vi "TestKeithley.vi"() -> ()   [LabVIEW 2017]
uses:
  <instrlib>/Keithley 24XX/Public/Data/Read (Measurements).vi
  <instrlib>/Keithley 24XX/Keithley 24XX.lvlib
panel:
  out "Waveform Chart 2":sgl[](graph)
  in  "stop":bool
  out "Current Measurements":sgl[](array[numeric])
  out "Timestamp Measurements":sgl[](array[numeric])
  in  "Keithley VISA":refnum<visa-resource-name>
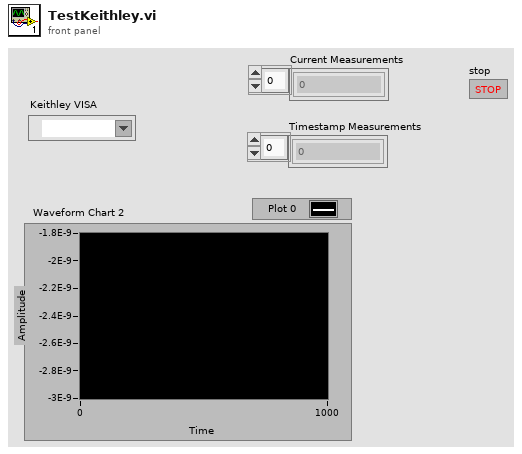
[diagram p1: front panel]
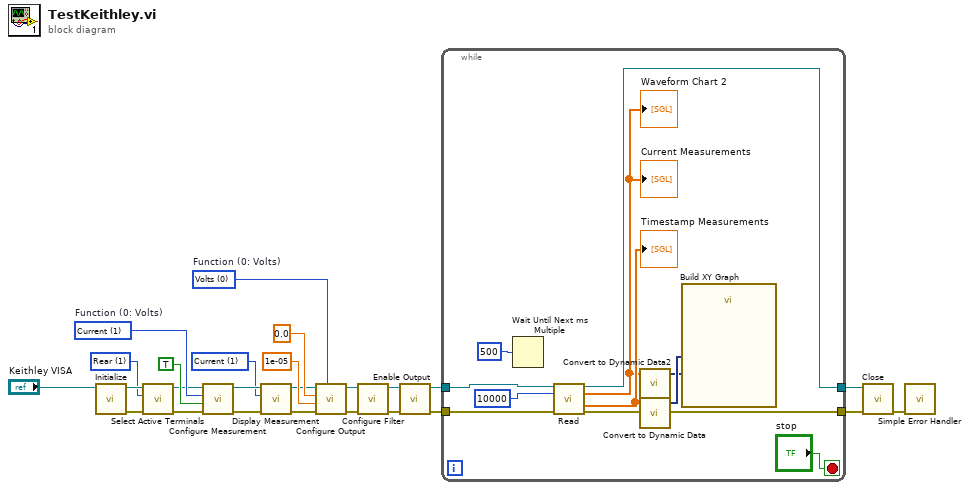
[diagram p0: block diagram]
diagram:
  w1 = u16 1 items=["Voltage", "Current", "Resistance"] ("Displayed Measurement (0: Voltage)")
  w14 = u16 1 items=["Front", "Rear"] ("Active Terminals (0: Front)")
  w19 = u16 0 items=["Volts", "Current", "Resistance"]  # Function (0: Volts)
  w23 = u16 1 items=["Volts", "Current", "Resistance"]  # Function (0: Volts)
  n1 = call <instrlib>:"Initialize.vi"("VISA resource name"="Keithley VISA") -> ("error out"=w15:errorcluster, "VISA resource name out"=w16:refnum<visa-resource-name>)  [unwired: 9 in]
  n2 = call <instrlib>:"Select Active Terminals.vi"("error in (no error)"=w15, "Active Terminals (0: Front)"=w14, "VISA resource name"=w16) -> ("error out"=w10:errorcluster, "VISA resource name out"=w11:refnum<visa-resource-name>)  [unwired: 7 in]
  n3 = call <instrlib>:"Configure Measurement.vi"("error in (no error)"=w10, "Enable Auto Range (T:Enable)"=TRUE, "Function (0: Volts)"=w23, "VISA resource name"=w11) -> ("error out"=w4:errorcluster, "VISA resource name out"=w5:refnum<visa-resource-name>)  [unwired: 6 in]
  n4 = call <instrlib>:"Display Measurement.vi"("error in (no error)"=w4, "Displayed Measurement (0: Voltage)"=w1, "VISA resource name"=w5) -> ("error out"=w3:errorcluster, "VISA resource name out"=w2:refnum<visa-resource-name>)  [unwired: 7 in]
  n5 = call <instrlib>:"Configure Output.vi"("Source Mode  (0: Voltage)"=w19, "error in (no error)"=w3, "Compliance  Level (0.1)"=1e-05, "Output Level (0)"=0.0, "VISA resource name"=w2) -> ("error out"=w6:errorcluster, "VISA resource name out"=w7:refnum<visa-resource-name>)  [unwired: 5 in]
  n6 = call <instrlib>:"Configure Filter.vi"("error in (no error)"=w6, "VISA resource name"=w7) -> ("error out"=w12:errorcluster, "VISA resource name out"=w13:refnum<visa-resource-name>)  [unwired: 8 in]
  n7 = call <instrlib>:"Enable Output.vi"("error in (no error)"=w12, "VISA resource name"=w13) -> ("error out"=w8:errorcluster, "VISA resource name out"=w9:refnum<visa-resource-name>)  [unwired: 8 in]
  n8 = while {
    tunnel: w9 -> [w34]
    tunnel: w8 -> [w33]
    tunnel: [w32] -> w21
    tunnel: [w31] -> w20
    stop <- "stop" stop-if-true
    n9 = Wait Until Next ms Multiple(millisecond multiple=u32 500) -> ()  [unwired: 1 out]
    n10 = call-poly <instrlib>:"Read.vi"("VISA resource name"=w34, "Timeout (10000 ms)"=10000, "error in (no error)"=w33) -> ("VISA resource name out"=w32:refnum<visa-resource-name>, "Current Measurements"=w26:sgl[], "Timestamp Measurements"=w28:sgl[], "error out"=w31:errorcluster)  [unwired: 6 in, 3 out]
    "Current Measurements" <- w26
    "Timestamp Measurements" <- w28
    "Waveform Chart 2" <- w26
    n11 = call "Convert to Dynamic Data2"("Array"=w26) -> ("Dynamic Data Type"=w35:dynamicdata)  [unwired: 3 in]
    n12 = call "Convert to Dynamic Data"("Array"=w28) -> ("Dynamic Data Type"=w36:dynamicdata)  [unwired: 3 in]
    n13 = call "Build XY Graph"("Y Input"=w35, "X Input"=w36) -> ()  [unwired: 8 in, 2 out]
  }
  n14 = call <instrlib>:"Close.vi"("error in (no error)"=w20, "VISA resource name"=w21) -> ("error out"=w22:errorcluster)  [unwired: 9 in]
  n15 = call <vilib>:"Simple Error Handler.vi"("error in (no error)"=w22) -> ()  [unwired: 4 in, 5 out]
